vi "objectcount.vi"() -> ()   [LabVIEW 2019]
panel:
  out "Array":i32[](array[numeric])
  out "size(s)":i32
  out "sum":i16
  in  "String":string
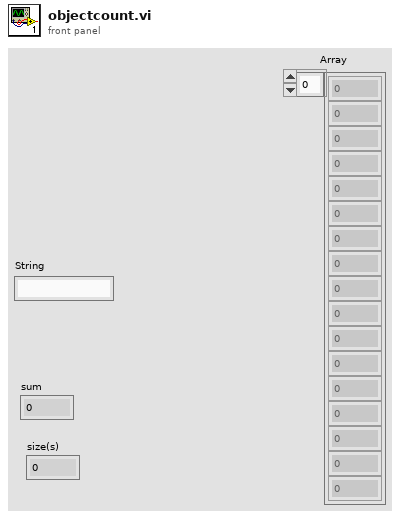
[diagram p1: front panel]
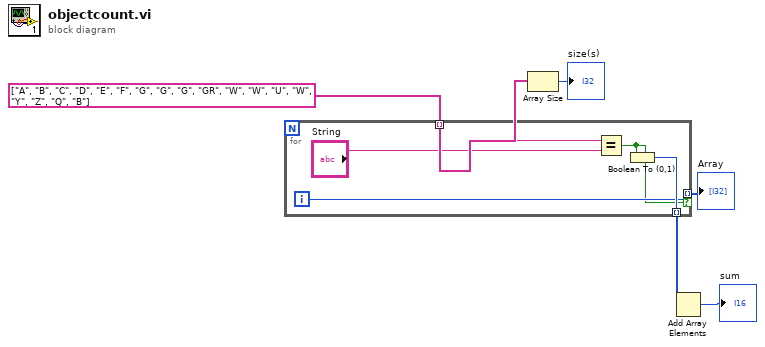
[diagram p0: block diagram]
diagram:
  w3 = string[] ["A", "B", "C", "D", "E", "F", "G", "G", "G", "GR", "W", "W", "U", "W", "Y", "Z", "Q", "B"]
  n1 = for {
    tunnel: [w9] -> w5 mode=indexing
    tunnel: w3 -> [w8] mode=indexing
    tunnel: [w7] -> w1 mode=indexing if=w6
    i -> [w7]
    n2 = Equal?(x=w8, y="String") -> (x = y?=w6:bool)
    n3 = Boolean To (0,1)(Boolean=w6) -> (0, 1=w9:i16)
  }
  "Array" <- w1
  n4 = Array Size(array=w3) -> (size(s)=→"size(s)":i32)
  n5 = Add Array Elements(numeric array=w5) -> (sum=→"sum":i16)
